vi "display_michelle_PKT_visjitter_stopadded_RandCont_PsuedoCO_FrameClock2.vi"() -> ()   [LabVIEW 2019]
uses:
  <vilib>/Analysis/Matrix/Datatypes/RealMatrix.ctl
  <vilib>/Utility/file.llb/Write Delimited Spreadsheet (DBL).vi
  <vilib>/Analysis/Matrix/NI_Matrix.lvlib
panel:
  out "lambda":dbl
  out "maxITI":dbl
  out "minITI":dbl
  out "goEXP":dbl
  out "meanITI":dbl
  out "ArrayTemp3":T1
  out "StimID2":dbl
  out "Contrast":dbl
  out "TimeOutCounter":i32
  out "ElapsedTime_M":dbl
  out "Base_Contrast":dbl
  out "CurrentTrial":u32=1
  out "Jitter":dbl
  out "BaseITI":dbl
  out "VisStimDuration":dbl
  in  "Stop":bool
  out "Num trials":u32=204
  out "ISI Time":dbl
  out "Stim TS":dbl
  out "Output":dbl[][](array[numeric])
  out "Output frame":T1
  out "Array temp1":T1
  out "Elapsed Time":dbl
  out "Display":bool=TRUE
  out "Trial":u32=1
  out "reward":dbl[](array[numeric])
  out "stim_id":dbl[](array[numeric])
  out "stim_loaded":dbl
  out "Timings":dbl[](array[numeric])
  out "Stimuli Loaded?":bool
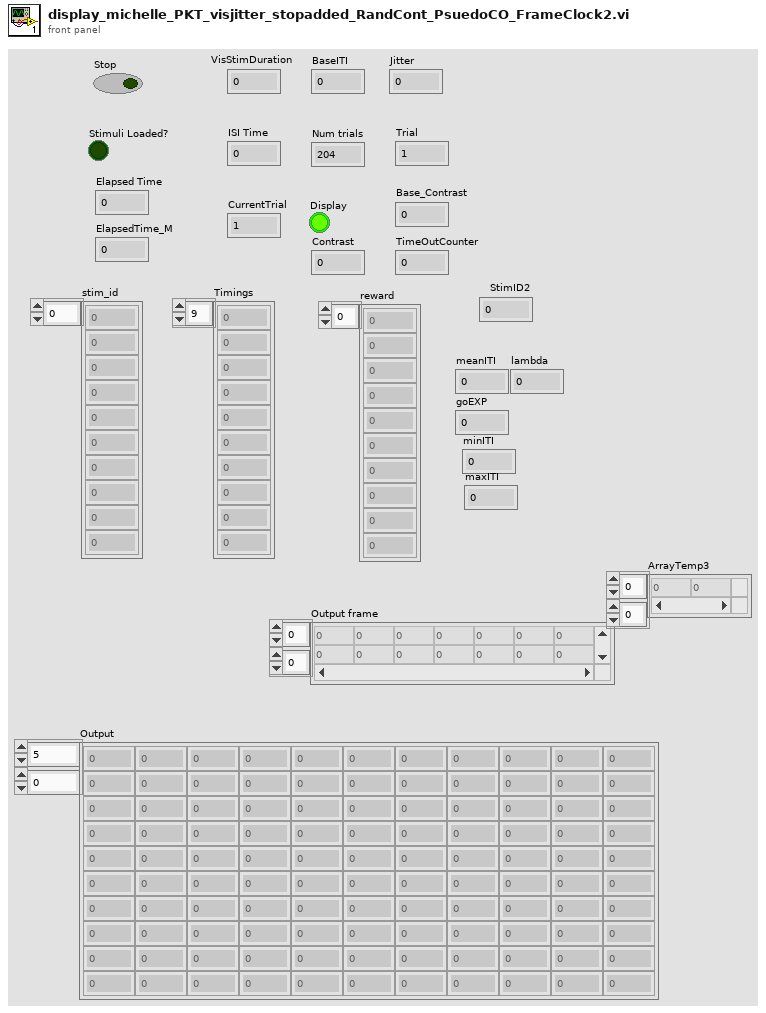
[diagram p1: front panel]
types:
  T1 = typedef "NI_Matrix.lvlib/RealMatrix.ctl" = dbl[][]
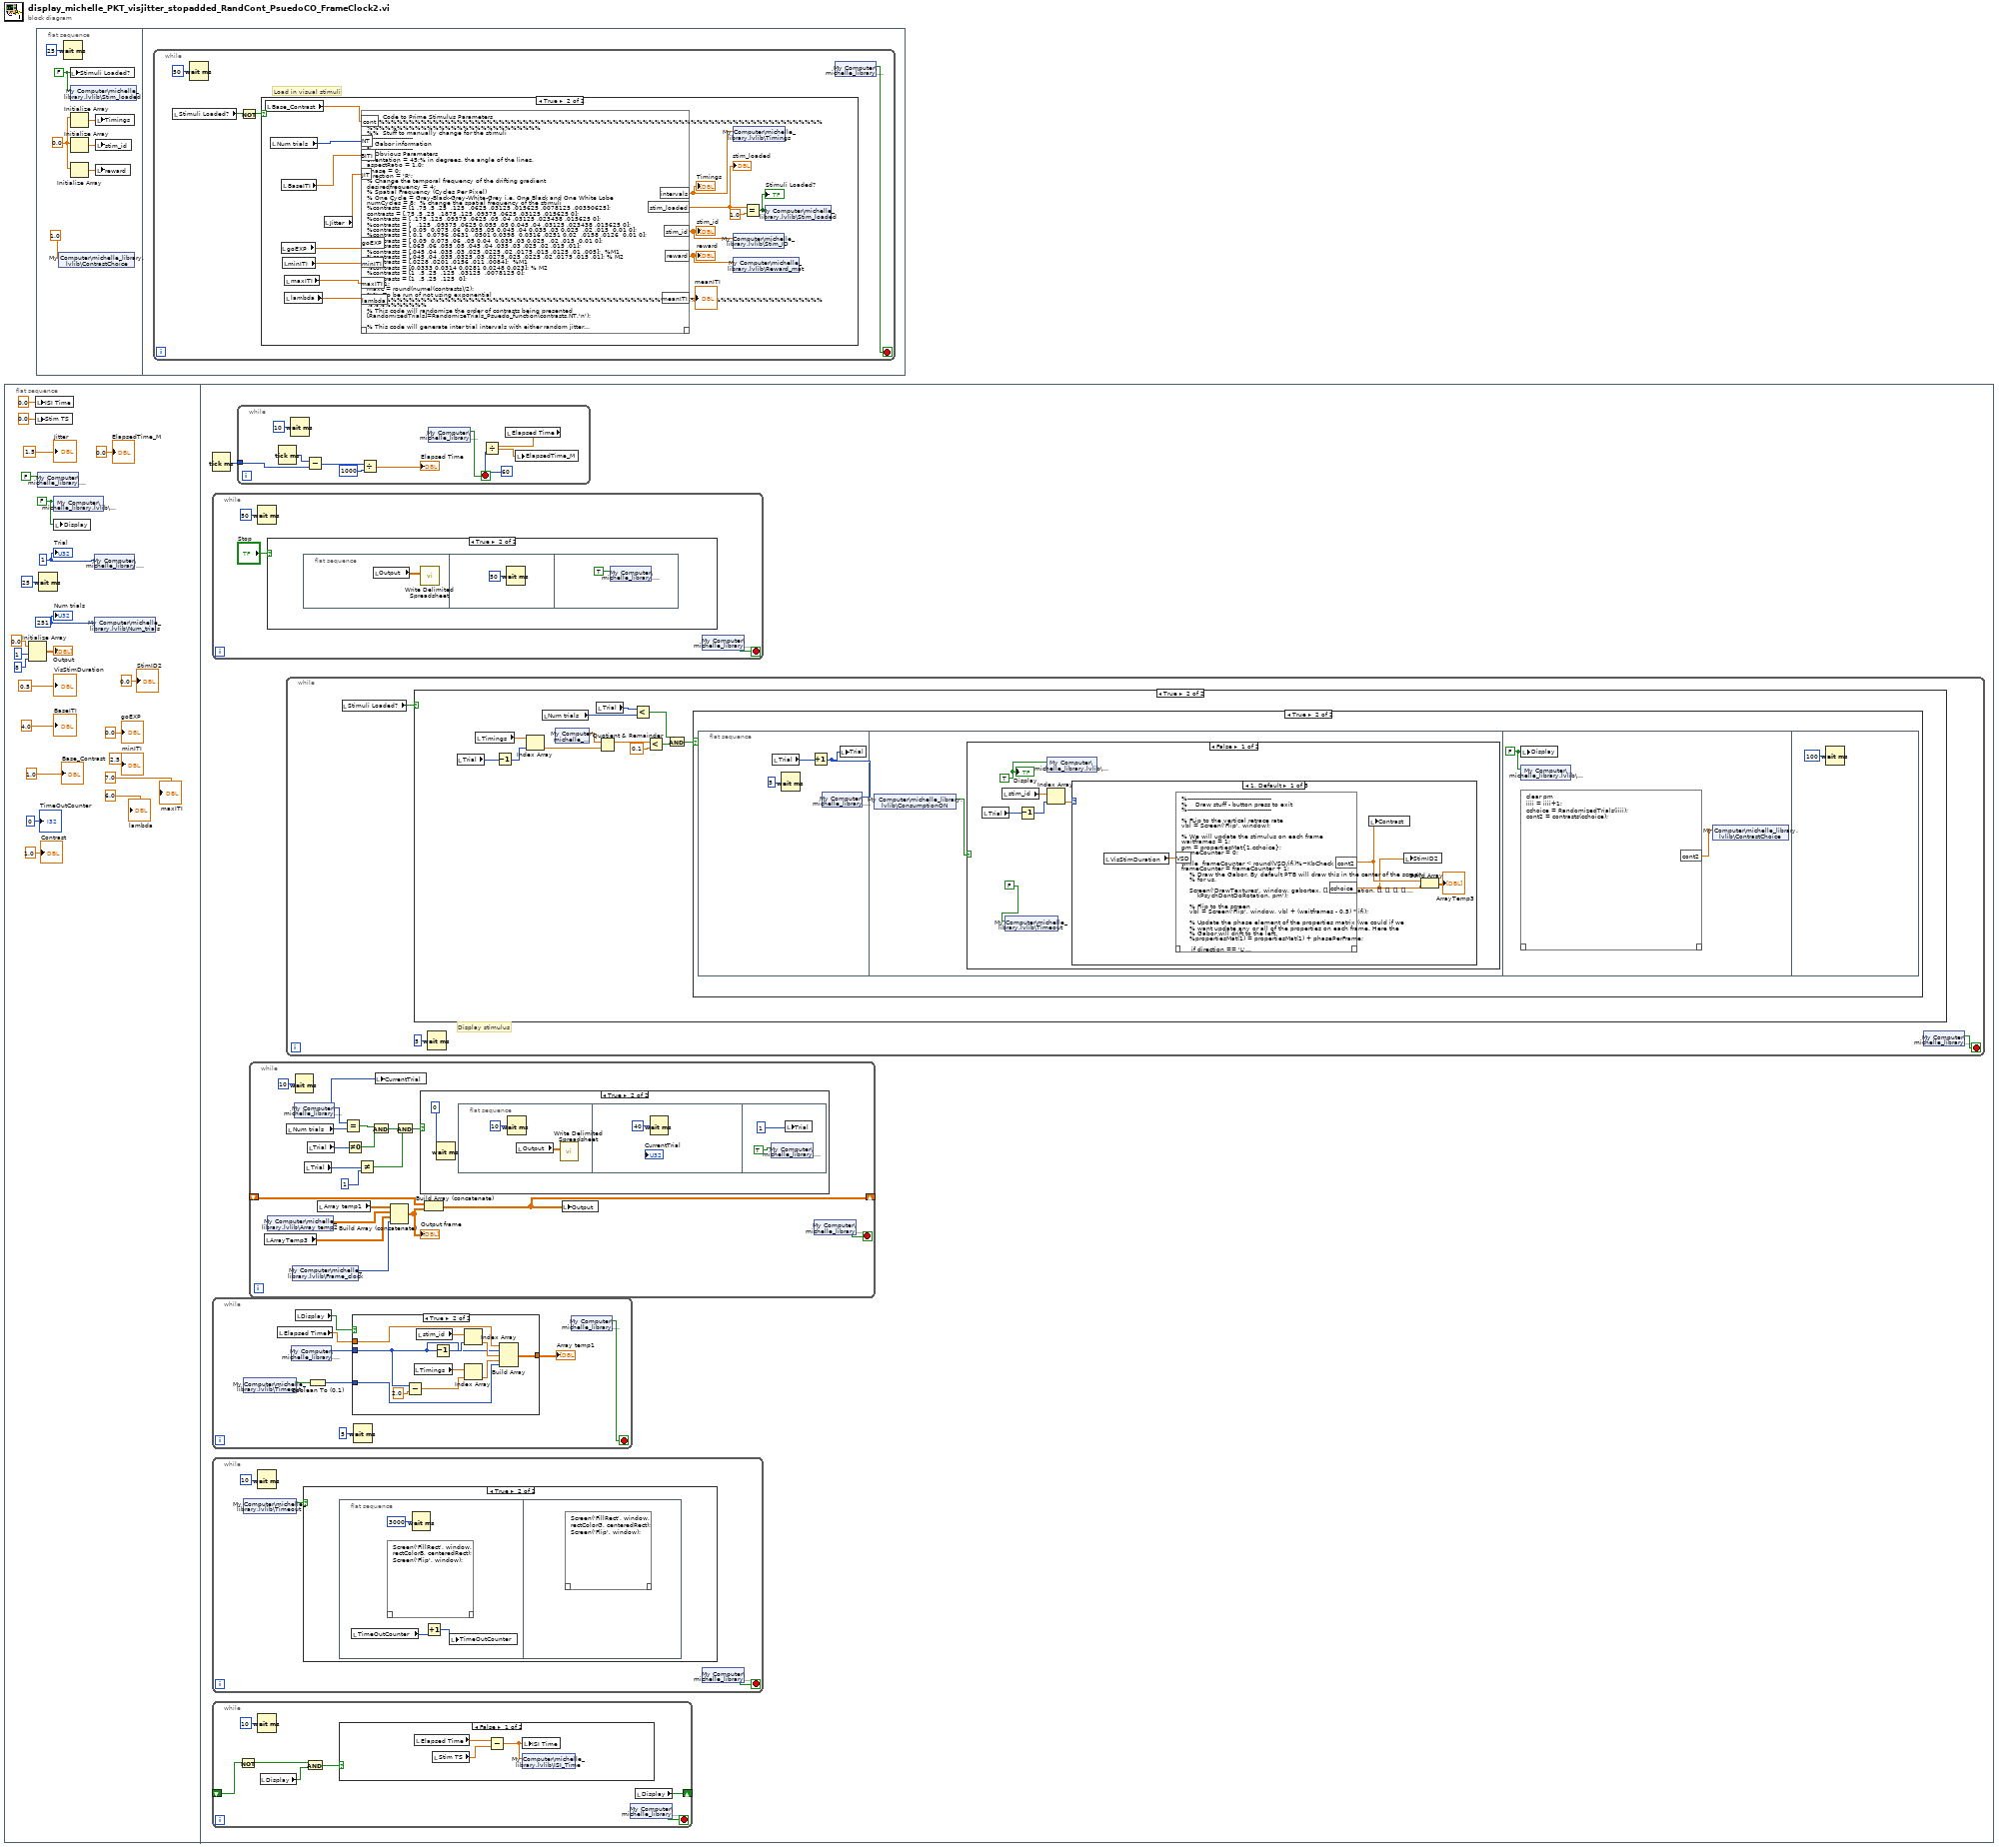
[diagram p0: block diagram]
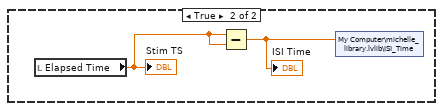
[diagram p5: hidden frame]
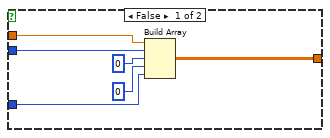
[diagram p6: hidden frame]
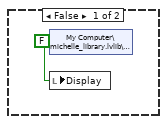
[diagram p9: hidden frame]
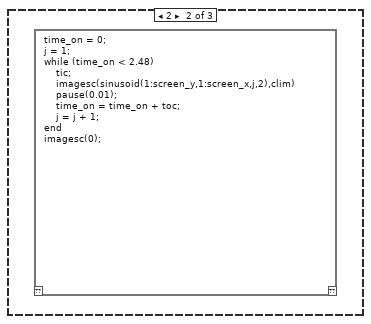
[diagram p10: hidden frame]
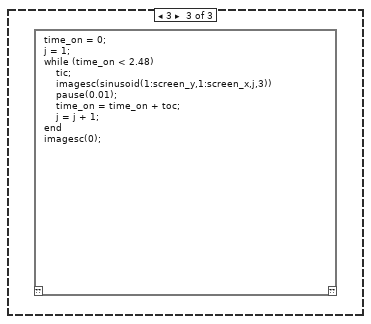
[diagram p11: hidden frame]
diagram:
  n1 = flat-sequence {
    frame #0 {
      w15 = u32 251
      w21 = FALSE ("Display")
      w23 = u32 1 ("Trial")
      n2 = Initialize Array(0.0 ("element"), 1 ("dimension size"), 8 ("dimension size")) -> (→"Output":dbl[][])
      n3 = local write "ISI Time"(0.0 ("ISI Time")) -> ()
      n4 = local write "Stim TS"(0.0 ("Stim TS")) -> ()
      n5 = shared-variable "My Computer\\michelle_library.lvlib\\Stop"(FALSE ("Stop")) -> ()  [unwired: 1 in, 1 out]
      n6 = Wait (ms)(milliseconds to wait=u32 25) -> ()  [unwired: 1 out]
      n7 = shared-variable "My Computer\\michelle_library.lvlib\\Display"(w21) -> ()  [unwired: 1 in, 1 out]
      n8 = local write "Display"(w21) -> ()
      n9 = shared-variable "My Computer\\michelle_library.lvlib\\Trial"(w23) -> ()  [unwired: 1 in, 1 out]
      n10 = shared-variable "My Computer\\michelle_library.lvlib\\Num_trials"(w15) -> ()  [unwired: 1 in, 1 out]
      "Trial" <- w23
      "Num trials" <- w15
      "VisStimDuration" <- 0.5
      "BaseITI" <- 4.0
      "Jitter" <- 1.5
      "Base_Contrast" <- 1.0
      "ElapsedTime_M" <- 0.0
      "TimeOutCounter" <- 0
      "Contrast" <- 1.0
      "StimID2" <- 0.0
      "goEXP" <- 0.0
      "minITI" <- 2.5
      "maxITI" <- 7.0
      "lambda" <- 6.0
    }
    frame #1 {
      n11 = Tick Count (ms)() -> (millisecond timer value=w24:u32)
      n12 = while {
        stop <- w27 stop-if-true
        n13 = Wait (ms)(milliseconds to wait=50) -> ()  [unwired: 1 out]
        n14 = case shown="True" "Stop" {
          frame False {
          }
          frame True {
            n15 = flat-sequence {
              frame #0 {
                n16 = local read "Output"() -> (w28:dbl[][])
                n17 = call-poly <vilib>:"Write Delimited Spreadsheet.vi"("2D data"=w28) -> ()  [unwired: 13 in, 2 out]
              }
              frame #1 {
                n18 = Wait (ms)(milliseconds to wait=50) -> ()  [unwired: 1 out]
              }
              frame #2 {
                n19 = shared-variable "My Computer\\michelle_library.lvlib\\Stop"(TRUE) -> ()  [unwired: 1 in, 1 out]
              }
            }
          }
        }
        n20 = shared-variable "My Computer\\michelle_library.lvlib\\Stop"() -> (w27:bool)  [unwired: 1 in, 1 out]
      }
      n21 = while {
        stop <- w51 stop-if-true
        n22 = shared-variable "My Computer\\michelle_library.lvlib\\Timeout"() -> (w49:bool)  [unwired: 1 in, 1 out]
        n23 = local read "Elapsed Time"() -> (w55:dbl)
        n24 = shared-variable "My Computer\\michelle_library.lvlib\\Trial"() -> (w53:u32)  [unwired: 1 in, 1 out]
        n25 = local read "Display"() -> (w52:bool)
        n26 = Boolean To (0,1)(Boolean=w49) -> (0, 1=w50:i16)
        n27 = case shown="True" w52 {
          tunnel: w53 -> [w61 w64]
          tunnel: w55 -> [w62 w71]
          tunnel: [w60 w72] -> w54
          tunnel: w50 -> [w57 w66]
          frame False {
            n28 = Build Array(w62, w61, u32 0 ("milliseconds to wait"), 0, w57) -> (w60:T1)
          }
          frame True {
            n29 = Subtract(x=w64, y=2.0) -> (x-y=w63:dbl)
            n30 = local read "Timings"() -> (w69:dbl[])
            n31 = local read "stim_id"() -> (w73:dbl[])
            n32 = Decrement(x=w64) -> (x-1=w68:u32)
            n33 = Index Array(array=w73, index=w68) -> (element=w70:dbl)
            n34 = Index Array(array=w69, index=w63) -> (element=w67:dbl)
            n35 = Build Array(w71, w64, w70, w67, w66) -> (w72:T1)
          }
        }
        "Array temp1" <- w54
        n36 = Wait (ms)(milliseconds to wait=u32 5) -> ()  [unwired: 1 out]
        n37 = shared-variable "My Computer\\michelle_library.lvlib\\Stop"() -> (w51:bool)  [unwired: 1 in, 1 out]
      }
      n38 = while {
        stop <- w33 stop-if-true
        n39 = shared-variable "My Computer\\michelle_library.lvlib\\Timeout"() -> (w31:bool)  [unwired: 1 in, 1 out]
        n40 = Wait (ms)(milliseconds to wait=u32 10) -> ()  [unwired: 1 out]
        n41 = case shown="True" w31 {
          frame False {
          }
          frame True {
            n42 = flat-sequence {
              frame #0 {
                n43 = local read "TimeOutCounter"() -> (w35:i32)
                n44 = script code="Screen('FillRect', window, rectColorB, centeredRect);\nScreen('Flip', window);"() -> ()  [unwired: 1 in, 1 out]
                n45 = Wait (ms)(milliseconds to wait=u32 3000) -> ()  [unwired: 1 out]
                n46 = Increment(x=w35) -> (x+1=w34:i32)
                n47 = local write "TimeOutCounter"(w34) -> ()
              }
              frame #1 {
                n48 = script code="Screen('FillRect', window, rectColorG, centeredRect);\nScreen('Flip', window);"() -> ()  [unwired: 1 in, 1 out]
              }
            }
          }
        }
        n49 = shared-variable "My Computer\\michelle_library.lvlib\\Stop"() -> (w33:bool)  [unwired: 1 in, 1 out]
      }
      n50 = while {
        shift-right: [w41] -> _
        shift-left: _ -> [w40]
        stop <- w43 stop-if-true
        n51 = Not(x=w40) -> (.not. x?=w39:bool)
        n52 = Wait (ms)(milliseconds to wait=u32 10) -> ()  [unwired: 1 out]
        n53 = local read "Display"() -> (w38:bool)
        n54 = And(x=w39, y=w38) -> (x .and. y?=w37:bool)
        n55 = case shown="False" w37 {
          frame False {
            n56 = local read "Elapsed Time"() -> (w44:dbl)
            n57 = local read "Stim TS"() -> (w46:dbl)
            n58 = Subtract(x=w44, y=w46) -> (x-y=w45:dbl)
            n59 = local write "ISI Time"(w45) -> ()
            n60 = shared-variable "My Computer\\michelle_library.lvlib\\ISI_Time"(w45) -> ()  [unwired: 1 in, 1 out]
          }
          frame True {
            n61 = local read "Elapsed Time"() -> (w47:dbl)
            "Stim TS" <- w47
            n62 = Subtract(x=w47, y=w47) -> (x-y=w48:dbl)
            "ISI Time" <- w48
            n63 = shared-variable "My Computer\\michelle_library.lvlib\\ISI_Time"(w48) -> ()  [unwired: 1 in, 1 out]
          }
        }
        n64 = shared-variable "My Computer\\michelle_library.lvlib\\Stop"() -> (w43:bool)  [unwired: 1 in, 1 out]
        n65 = local read "Display"() -> (w41:bool)
      }
      n66 = while {
        tunnel: w24 -> [w80]
        stop <- w77 stop-if-true
        n67 = Tick Count (ms)() -> (millisecond timer value=w81:u32)
        n68 = Wait (ms)(milliseconds to wait=u32 10) -> ()  [unwired: 1 out]
        n69 = Subtract(x=w81, y=w80) -> (x-y=w78:u32)
        n70 = Divide(x=w78, y=u32 1000) -> (x/y=→"Elapsed Time":dbl)
        n71 = shared-variable "My Computer\\michelle_library.lvlib\\Stop"() -> (w77:bool)  [unwired: 1 in, 1 out]
        n72 = local read "Elapsed Time"() -> (w74:dbl)
        n73 = Divide(x=w74, y=60) -> (x/y=w76:dbl)
        n74 = local write "ElapsedTime_M"(w76) -> ()
      }
      n75 = while {
        shift-right: [w99] -> _
        shift-left: _ -> [w100]
        stop <- w102 stop-if-true
        n76 = local read "ArrayTemp3"() -> (w85:T1)
        n77 = shared-variable "My Computer\\michelle_library.lvlib\\Array temp2"() -> (w97:dbl[][])  [unwired: 1 in, 1 out]
        n78 = local read "Num trials"() -> (w95:u32)
        n79 = shared-variable "My Computer\\michelle_library.lvlib\\Frame_clock"() -> (w84:u32)  [unwired: 1 in, 1 out]
        n80 = shared-variable "My Computer\\michelle_library.lvlib\\Trial"() -> (w86:u32)  [unwired: 1 in, 1 out]
        n81 = Wait (ms)(milliseconds to wait=u32 10) -> ()  [unwired: 1 out]
        n82 = local read "Trial"() -> (w92:u32)
        n83 = local read "Trial"() -> (w93:u32)
        n84 = local read "Array temp1"() -> (w98:T1)
        n85 = Equal?(x=w86, y=w95) -> (x = y?=w94:bool)
        n86 = Not Equal To 0?(x=w93) -> (x != 0?=w89:bool)
        n87 = Not Equal?(x=w92, y=1) -> (x != y?=w91:bool)
        n88 = And(x=w94, y=w89) -> (x .and. y?=w87:bool)
        n89 = local write "CurrentTrial"(w86) -> ()
        n90 = Build Array (concatenate)(w98, w97, w85, w84) -> (w96:T1)
        "Output frame" <- w96
        n91 = And(x=w87, y=w91) -> (x .and. y?=w88:bool)
        n92 = case shown="True" w88 {
          frame False {
          }
          frame True {
            n93 = Wait (ms)(milliseconds to wait=0) -> ()  [unwired: 1 out]
            n94 = flat-sequence {
              frame #0 {
                n95 = Wait (ms)(milliseconds to wait=u32 10) -> ()  [unwired: 1 out]
                n96 = local read "Output"() -> (w105:dbl[][])
                n97 = call-poly <vilib>:"Write Delimited Spreadsheet.vi"("2D data"=w105) -> ()  [unwired: 13 in, 2 out]
              }
              frame #1 {
                n98 = Wait (ms)(milliseconds to wait=u32 40) -> ()  [unwired: 1 out]
              }
              frame #2 {
                n99 = shared-variable "My Computer\\michelle_library.lvlib\\Stop"(TRUE) -> ()  [unwired: 1 in, 1 out]
                n100 = local write "Trial"(1) -> ()
              }
            }
          }
        }
        n101 = Build Array (concatenate) ("Build Matrix")(w100, w96) -> (w99:T1)
        n102 = local write "Output"(w99) -> ()
        n103 = shared-variable "My Computer\\michelle_library.lvlib\\Stop"() -> (w102:bool)  [unwired: 1 in, 1 out]
      }
      n104 = while {
        stop <- w110 stop-if-true
        # "Display stimulus"
        n105 = local read "Stimuli Loaded?"() -> (w109:bool)
        n106 = case shown="True" w109 {
          frame False {
          }
          frame True {
            n107 = local read "Trial"() -> (w112:u32)
            n108 = local read "Timings"() -> (w121:dbl[])
            n109 = Decrement(x=w112) -> (x-1=w113:u32)
            n110 = Index Array(array=w121, index=w113) -> (element=w120:dbl)
            n111 = local read "Num trials"() -> (w116:u32)
            n112 = shared-variable "My Computer\\michelle_library.lvlib\\ISI"() -> (w115:dbl)  [unwired: 1 in, 1 out]
            n113 = local read "Trial"() -> (w119:u32)
            n114 = Quotient & Remainder(x=w115, y=w120) -> (x-y*floor(x/y)=w123:dbl)  [unwired: 1 out]
            n115 = Less?(x=w119, y=w116) -> (x < y?=w118:bool)
            n116 = Less?(x=w123, y=0.1) -> (x < y?=w117:bool)
            n117 = And(x=w118, y=w117) -> (x .and. y?=w114:bool)
            n118 = case shown="True" w114 {
              frame False {
                w124 = FALSE ("Display")
                n119 = shared-variable "My Computer\\michelle_library.lvlib\\Display"(w124) -> ()  [unwired: 1 in, 1 out]
                n120 = local write "Display"(w124) -> ()
              }
              frame True {
                n121 = flat-sequence {
                  frame #0 {
                    n122 = local read "Trial"() -> (w127:u32)
                    n123 = Wait (ms)(milliseconds to wait=u32 5) -> ()  [unwired: 1 out]
                    n124 = Increment(x=w127) -> (x+1=w126:u32)
                    n125 = shared-variable "My Computer\\michelle_library.lvlib\\Trial"(w126) -> ()  [unwired: 1 in, 1 out]
                    n126 = local write "Trial"(w126) -> ()
                  }
                  frame #1 {
                    n127 = shared-variable "My Computer\\michelle_library.lvlib\\ConsumptionON"() -> (w128:bool)  [unwired: 1 in, 1 out]
                    n128 = case shown="False" w128 {
                      frame False {
                        w129 = TRUE ("Boolean")
                        n129 = local read "Trial"() -> (w132:u32)
                        n130 = local read "stim_id"() -> (w134:dbl[])
                        n131 = shared-variable "My Computer\\michelle_library.lvlib\\Timeout"(FALSE) -> ()  [unwired: 1 in, 1 out]
                        n132 = Decrement(x=w132) -> (x-1=w131:u32)
                        n133 = shared-variable "My Computer\\michelle_library.lvlib\\Display"(w129) -> ()  [unwired: 1 in, 1 out]
                        n134 = Index Array(array=w134, index=w131) -> (element=w133:dbl)
                        n135 = case shown="1, Default" w133 {
                          frame 1, Default {
                            n136 = local read "VisStimDuration"() -> (w138:dbl)
                            n137 = script code="%------------------------------------------\n%    Draw stuff - button press to exit\n%------------------------------------------\n\n% FLip to the vertical retrace rate\nvbl = Screen('Flip', window);\n\n% We will update the stimulus on each frame\nwaitframes = 1;\npm = propertiesMat{1,cchoice};\nframeCounter = 0;\ntic\nwhile  frameCounter < round(VSD/ifi)%~KbCheck\nframeCounter = frameCounter + 1;\n    % Draw the Gabor. By default PTB will draw this in the center of the screen\n    % for us.\n   \n    Screen('DrawTextures', window, gabortex, [], [], orientation, [], [], [], [],...\n        kPsychDontDoRotation, pm');\n\n    % Flip to the screen\n    vbl = Screen('Flip', window, vbl + (waitframes - 0.5) * ifi);\n\n    % Update the phase element of the properties matrix (we could if we\n    % want update any or all of the properties on each frame. Here the\n    % Gabor will drift to the left.\n    %propertiesMat(1) = propertiesMat(1) + phasePerFrame;\n \n     if direction == 'L'\n          pm(1) = pm(1) + phasePerFrame;\n     elseif direction =='R'\n          pm(1) = pm(1) - phasePerFrame;\n     end\n\nend\nTime(N) = toc;\nvbl = Screen('Flip', window);"("VSD"=w138) -> ("cont2"=w137:dbl, "cchoice"=w136:dbl)  [unwired: 1 in, 1 out]
                            n138 = local write "Contrast"(w137) -> ()
                            n139 = local write "StimID2"(w136) -> ()
                            n140 = Build Array(w137, w136) -> (→"ArrayTemp3":T1)
                          }
                          frame 2 {
                            n141 = script code="time_on = 0;\nj = 1;\nwhile (time_on < 2.48)\n    tic;\n    imagesc(sinusoid(1:screen_y,1:screen_x,j,2),clim)\n    pause(0.01);\n    time_on = time_on + toc;\n    j = j + 1;\nend\nimagesc(0);"() -> ()  [unwired: 1 in, 1 out]
                          }
                          frame 3 {
                            n142 = script code="time_on = 0;\nj = 1;\nwhile (time_on < 2.48)\n    tic;\n    imagesc(sinusoid(1:screen_y,1:screen_x,j,3))\n    pause(0.01);\n    time_on = time_on + toc;\n    j = j + 1;\nend\nimagesc(0);"() -> ()  [unwired: 1 in, 1 out]
                          }
                        }
                        "Display" <- w129
                      }
                      frame True {
                      }
                    }
                  }
                  frame #2 {
                    w140 = FALSE ("Display")
                    n143 = script code="clear pm\niiii = iiii+1;\ncchoice = RandomizedTrials(iiii);\ncont2 = contrasts(cchoice);"() -> ("cont2"=w139:dbl)  [unwired: 1 in, 1 out]
                    n144 = local write "Display"(w140) -> ()
                    n145 = shared-variable "My Computer\\michelle_library.lvlib\\Display"(w140) -> ()  [unwired: 1 in, 1 out]
                    n146 = shared-variable "My Computer\\michelle_library.lvlib\\ContrastChoice"(w139) -> ()  [unwired: 1 in, 1 out]
                  }
                  frame #3 {
                    n147 = Wait (ms)(milliseconds to wait=u32 100) -> ()  [unwired: 1 out]
                  }
                }
              }
            }
          }
        }
        n148 = Wait (ms)(milliseconds to wait=u32 5) -> ()  [unwired: 1 out]
        n149 = shared-variable "My Computer\\michelle_library.lvlib\\Stop"() -> (w110:bool)  [unwired: 1 in, 1 out]
      }
    }
  }
  n150 = flat-sequence {
    frame #0 {
      w145 = 0.0 ("element")
      w143 = FALSE ("Stimuli Loaded?")
      n151 = shared-variable "My Computer\\michelle_library.lvlib\\ContrastChoice"(1.0) -> ()  [unwired: 1 in, 1 out]
      n152 = Wait (ms)(milliseconds to wait=u32 25) -> ()  [unwired: 1 out]
      n153 = local write "Stimuli Loaded?"(w143) -> ()
      n154 = shared-variable "My Computer\\michelle_library.lvlib\\Stim_loaded"(w143) -> ()  [unwired: 1 in, 1 out]
      n155 = Initialize Array(w145) -> (w147:dbl[])  [unwired: 1 in]
      n156 = Initialize Array(w145) -> (w146:dbl[])  [unwired: 1 in]
      n157 = Initialize Array(w145) -> (w144:dbl[])  [unwired: 1 in]
      n158 = local write "Timings"(w147) -> ()
      n159 = local write "stim_id"(w146) -> ()
      n160 = local write "reward"(w144) -> ()
    }
    frame #1 {
      n161 = while {
        stop <- w151 stop-if-true
        # "Load in visual stimuli"
        n162 = local read "Stimuli Loaded?"() -> (w150:bool)
        n163 = Wait (ms)(milliseconds to wait=u32 50) -> ()  [unwired: 1 out]
        n164 = Not(x=w150) -> (.not. x?=w149:bool)
        n165 = case shown="True" w149 {
          frame False {
          }
          frame True {
            n166 = local read "Base_Contrast"() -> (w158:dbl)
            n167 = local read "Num trials"() -> (w161:u32)
            n168 = local read "goEXP"() -> (w154:dbl)
            n169 = local read "BaseITI"() -> (w160:dbl)
            n170 = local read "minITI"() -> (w155:dbl)
            n171 = local read "maxITI"() -> (w156:dbl)
            n172 = local read "lambda"() -> (w157:dbl)
            n173 = local read "Jitter"() -> (w159:dbl)
            n174 = script code="%%  Code to Prime Stimulus Parameters\n%%%%%%%%%%%%%%%%%%%%%%%%%%%%%%%%%%%%%%%%%%%%%%%%%%%%%%%%%%%%%%%%%%%%%%%%%%%%%%%%%%%%%%%%%%%%%%%%%%%%%%%%%\n%%  Stuff to manually change for the stimuli\n%--------------------\n% Gabor information\n%--------------------\n% Obvious Parameters\norientation = 45;% in degrees, the angle of the lines.\naspectRatio = 1.0;\nphase = 0;\ndirection = 'R';\n% Change the temporal frequency of the drifting gradient\ndesiredfrequency = 4;\n% Spatial Frequency (Cycles Per Pixel)\n% One Cycle = Grey-Black-Grey-White-Grey i.e. One Black and One White Lobe\nnumCycles = 8;  % change the spatial frequency of the stimuli\n%contrasts = [1 .75 .5 .25  .125  .0625 .03125 .015625 .0078125 .00390625];\ncontrasts = [.75 .5 .25  .1875 .125 .09375 .0625 .03125 .015625 0];\n%contrasts = [ .175 .125 .09375 .0625 .05 .04 .03125 .023438 .015625 0];\n%contrasts = [   .125  .09375 .0625 0.055 .05 0.045 .04 .03125 .023438 .015625 0];\n%contrasts = [ 0.09  0.075 .06  0.055 .05 0.045 .04 0.035 .03 0.025  .02 .015  0.01 0];\n%contrasts = [ 0.1  0.0796 .0631  .0501 0.0398  0.0316 .0251 0.02  .0158 .0126  0.01 0];\n%contrasts = [ 0.09  0.075 .06  .05 0.04  0.035 .03 0.025  .02 .015  0.01 0];\n%contrasts = [.065 .06 .055 .05 .045 .04 .035 .03 .025 .02 .015 .01];\n%contrasts = [.045 .04 .035 .03 .025 .0225 .02 .0175 .015 .0125 .01 .005];  %M1\n%contrasts = [.045 .04 .035 .0325 .03 .0275 .025 .0225 .02 .0175 .015 .01]; % M2\n%contrasts = [.0228 .0201 .0156 .011 .0084];  %M1\n%contrasts = [0.0333 0.0314 0.0281 0.0248 0.023]; % M2\n%contrasts = [1  .5 .25  .125  .03125  .0078125 0];\n%contrasts = [1  .5 .25  .125  0];\ngo = 1;\nmaxc = round(numel(contrasts)/2);\n%%  To be run of not using exponential\n%%%%%%%%%%%%%%%%%%%%%%%%%%%%%%%%%%%%%%%%%%%%%%%%%%%%%%%%%%%%%%%%%%%%%%%%%%%%%%%%%%%%%%\n% This code will randomize the order of contrasts being presented\n[RandomizedTrials]=RandomizeTrials_Psuedo_function(contrasts,NT,'n');\n\n% This code will generate inter trial intervals with either random jitter\n% or based on an exponential distribution\nif goEXP < 1\n     jit = JIT;\n     jitter = rand(1,NT);\n     jitter = 2*jit*(jitter- .5);\n     ITIbase = BITI;\n     intervals = [ones(1,NT)*ITIbase];\n     intervals = intervals + jitter;\nelseif goEXP > 0\n     intervals = exponentialITI(1/lambda, minITI, maxITI, NT);\nend\n\n%%  Prep the stimulus presentation software\n%%%%%%%%%%%%%%%%%%%%%%%%%%%%%%%%%%%%%%%%%%%%%%%%%%%%%%%%%%%%%%%%%%%%%%%%%%%\n%Screen('Preference', 'SkipSyncTests', 1);\nsca;\nclose all;\n% Setup PTB with some default values\nPsychDefaultSetup(2);\n% Set the screen number to the external secondary monitor if there is one connected\nscreenNumber = max(Screen('Screens'));\n\n% Define black, white and grey\nwhite = WhiteIndex(screenNumber);\nblack = BlackIndex(screenNumber);\ngrey = white / 2;\n\n% Open the screen & define it's dimensions\n[window, windowRect] = PsychImaging('OpenWindow', screenNumber, grey,...\n    [], 32, 2, [], [], kPsychNeedRetinaResolution);\n[screenXpixels, screenYpixels] = Screen('WindowSize', window);\n[xCenter, yCenter] = RectCenter(windowRect);\n\n% Get the vertical refresh rate of the monitor\nifi = Screen('GetFlipInterval', window);\n\n% Set maximum priority level\ntopPriorityLevel = MaxPriority(window);\nPriority(topPriorityLevel);\n\n\n% Build a procedural gabor texture (Note: to get a \"standard\" Gabor patch\n% we set a grey background offset, disable normalisation, and set a\n% pre-contrast multiplier of 0.5).\n% Dimension of the region where will draw the Gabor in pixels\ngaborDimPix = windowRect(3);\n% Sigma of Gaussian  (how much to fade around the edges)\nsigma = gaborDimPix / 0;  % change the 0 value to alter the fading\nphasePerFrame = desiredfrequency*360*ifi;\nfreq = numCycles / gaborDimPix;\n\nbackgroundOffset = [0.5 0.5 0.5 0.0];\ndisableNorm = 1;\npreContrastMultiplier = 0.5;\ngabortex = CreateProceduralGabor(window, gaborDimPix, gaborDimPix, [],...\n    backgroundOffset, disableNorm, preContrastMultiplier);\n\n% Randomise the phase of the Gabors and make a properties matrix.\nfor N = 1:numel(contrasts)\npropertiesMat{1,N} = [phase, freq, sigma, contrasts(N), aspectRatio, 0, 0, 0];\nend\n\niiii = 1;\ncchoice = RandomizedTrials(iiii);\ncont2 = contrasts(cchoice);\npm = propertiesMat{1,1};\n\n\n%%  Build up the rectangles for the pause and hold screen\nbaseRect = [0 0 screenXpixels screenYpixels];\ncenteredRect = CenterRectOnPointd(baseRect, xCenter, yCenter);\nrectColorB = [0 0 0];\nrectColorG = [128 128 128]/255;\n\n%%  Finalize the trial data and orders\nstim_id = [ones(1,NT)*1];\nreward = [ones(1,NT)*1];\nmeanITI = nanmean(intervals);\nrand_idx1 = randperm(NT);\nrand_idx2 = randperm(NT);\nintervals = intervals(rand_idx2);\nstim_id = stim_id(rand_idx2);\nreward = reward(rand_idx2);\n%%  All Done!\n%  indicate that the necessary preloading of data has been completed.\nstim_loaded = 1;" ("Script Node")("NT"=w161, "BITI"=w160, "JIT"=w159, "cont"=w158, "goEXP"=w154, "minITI"=w155, "maxITI"=w156, "lambda"=w157) -> ("stim_loaded"=w167:dbl, "intervals"=w162:dbl[], "stim_id"=w163:dbl[], "reward"=w165:dbl[], "meanITI"=→"meanITI":dbl)  [unwired: 1 in, 1 out]
            "stim_loaded" <- w167
            "Timings" <- w162
            "stim_id" <- w163
            "reward" <- w165
            n175 = shared-variable "My Computer\\michelle_library.lvlib\\Timings"(w162) -> ()  [unwired: 1 in, 1 out]
            n176 = shared-variable "My Computer\\michelle_library.lvlib\\Stim_ID"(w163) -> ()  [unwired: 1 in, 1 out]
            n177 = shared-variable "My Computer\\michelle_library.lvlib\\Reward_mat"(w165) -> ()  [unwired: 1 in, 1 out]
            n178 = Equal?(x=w167, y=1.0) -> (x = y?=w164:bool)
            "Stimuli Loaded?" <- w164
            n179 = shared-variable "My Computer\\michelle_library.lvlib\\Stim_loaded"(w164) -> ()  [unwired: 1 in, 1 out]
          }
        }
        n180 = shared-variable "My Computer\\michelle_library.lvlib\\Stop"() -> (w151:bool)  [unwired: 1 in, 1 out]
      }
    }
  }
